vi "DriveControlLoop.vi"() -> ()   [LabVIEW 2018]
uses:
  <vilib>/Rock Robotics/WPI/ThirdParty/Phoenix-LabVIEW/Motor Controller/Controls/CTRE_Phoenix_MotorControl_ControlMode.ctl
  Infrastructure/RobotMap.vi
  Robot Global Data.vi
  <vilib>/Rock Robotics/WPI/ThirdParty/Phoenix-LabVIEW/Motor Controller/Get/CTRE_Phoenix_MotorController_GetQuadratureData.vi
panel:
  out "Motor Outupt":dbl[](graph)
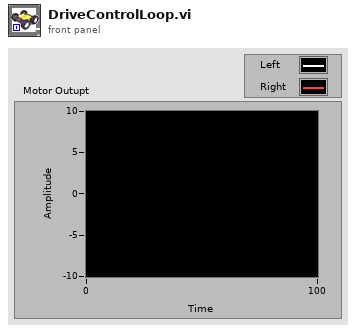
[diagram p1: front panel]
types:
  T1 = typedef "CTRE_Phoenix_MotorControl_ControlMode.ctl" = u16
  T2 = typedef "WPI_MotorControlDeviceRef.ctl" = cluster{"DeviceStatus":errorcluster, "Type":T3, "PWM":cluster{"PWM Channel":T4, "DeadBand":T5}, "CAN":cluster{"Device Number":u8, "SetOutput VI Ref":variant, "GetOutput VI Ref":variant, "Enable VI Ref":variant, "Disable VI Ref":variant, "Data":variant}, "Invert":bool, "DIO PWM":cluster{"PWM \"Enable\" Channel":T4, "DIOChannel":T6, "PWM Rate":dbl}}
  T3 = typedef "WPI_MotorControlType.ctl" = enum16{"PWM", "CAN", "DIO PWM"}
  T4 = typedef "FPGA_DIOPWMChannel.ctl" = enum8{"PWM 0", "PWM 1", "PWM 2", "PWM 3", "PWM 4", "PWM 5", "PWM 6", "PWM 7", "PWM 8", "PWM 9", "PWM MXP 0", "PWM MXP 1", "PWM MXP 2", "PWM MXP 3", "PWM MXP 4", "PWM MXP 5", "PWM MXP 6", "PWM MXP 7", "PWM MXP 8", "PWM MXP 9", "Invalid"}
  T5 = typedef "WPI_PWMDeadband.ctl" = cluster{"Name":string, "maxPositivePwm":i32, "minPositivePwm":i32, "centerPwm":i32, "maxNegativePwm":i32, "minNegativePwm":i32, "angularRange":u16}
  T6 = typedef "FPGA_DIOChannel.ctl" = enum8{"DIO 0", "DIO 1", "DIO 2", "DIO 3", "DIO 4", "DIO 5", "DIO 6", "DIO 7", "DIO 8", "DIO 9", "DIO MXP 0", "DIO MXP 1", "DIO MXP 2", "DIO MXP 3", "DIO MXP 4", "DIO MXP 5", "DIO MXP 6", "DIO MXP 7", "DIO MXP 8", "DIO MXP 9", "DIO MXP 10", "DIO MXP 11", "DIO MXP 12", "DIO MXP 13", "DIO MXP 14", "DIO MXP 15", "SPI Port CS1", "SPI Port CS2", "SPI Port CS3", "SPI Port MISO", "SPI Port MOSI", "Invalid"}
  T7 = typedef "WPI_DriverStationRobotMode2.ctl" = enum16{"Autonomous Disabled", "Autonomous Enabled", "Teleop Disabled", "Teleop Enabled", "Disconnected", "Finish", "Test Disabled", "Test Enabled", "Emergency Stopped"}
  T8 = typedef "Drive Motion Magic Setpoints.ctl" = cluster{"Increase in Left":dbl, "Increase in Right":dbl}[]
  T9 = cluster{"Increase in Left":dbl, "Increase in Right":dbl}
  T10 = typedef "Joystick Controls.ctl" = cluster{"Driver Left Joystick X":dbl, "Driver Left Joystick Y":dbl, "Driver A Button":bool, "Driver B Button":bool, "Driver X Button":bool, "Driver Y Button":bool, "Driver Left Bumper":bool, "Driver Right Bumper":bool, "Driver View Button":bool, "Driver Menu Button":bool, "Driver Left Joystick Press":bool, "Driver Right Joystick Press":bool, "Driver Left Trigger":dbl, "Driver Right Joystick X":dbl, "Driver Right Joystick Y":dbl, "Driver Right Trigger":dbl, "Operator Left Joystick X":dbl, "Operator Left Joystick Y":dbl, "Operator A Button":bool, "Operator B Button":bool, "Operator X Button":bool, "Operator Y Button":bool, "Operator Left Bumper":bool, "Operator Right Bumper":bool, "Operator View Button":bool, "Operator Menu Button":bool, "Operator Left Joystick Press":bool, "Operator Right Joystick Press":bool, "Operator Left Trigger":dbl, "Operator Right Joystick X":dbl, "Operator Right Joystick Y":dbl, "Operator Right Trigger":dbl, "Driver D-Pad":i16, "Operator D-Pad":i16}
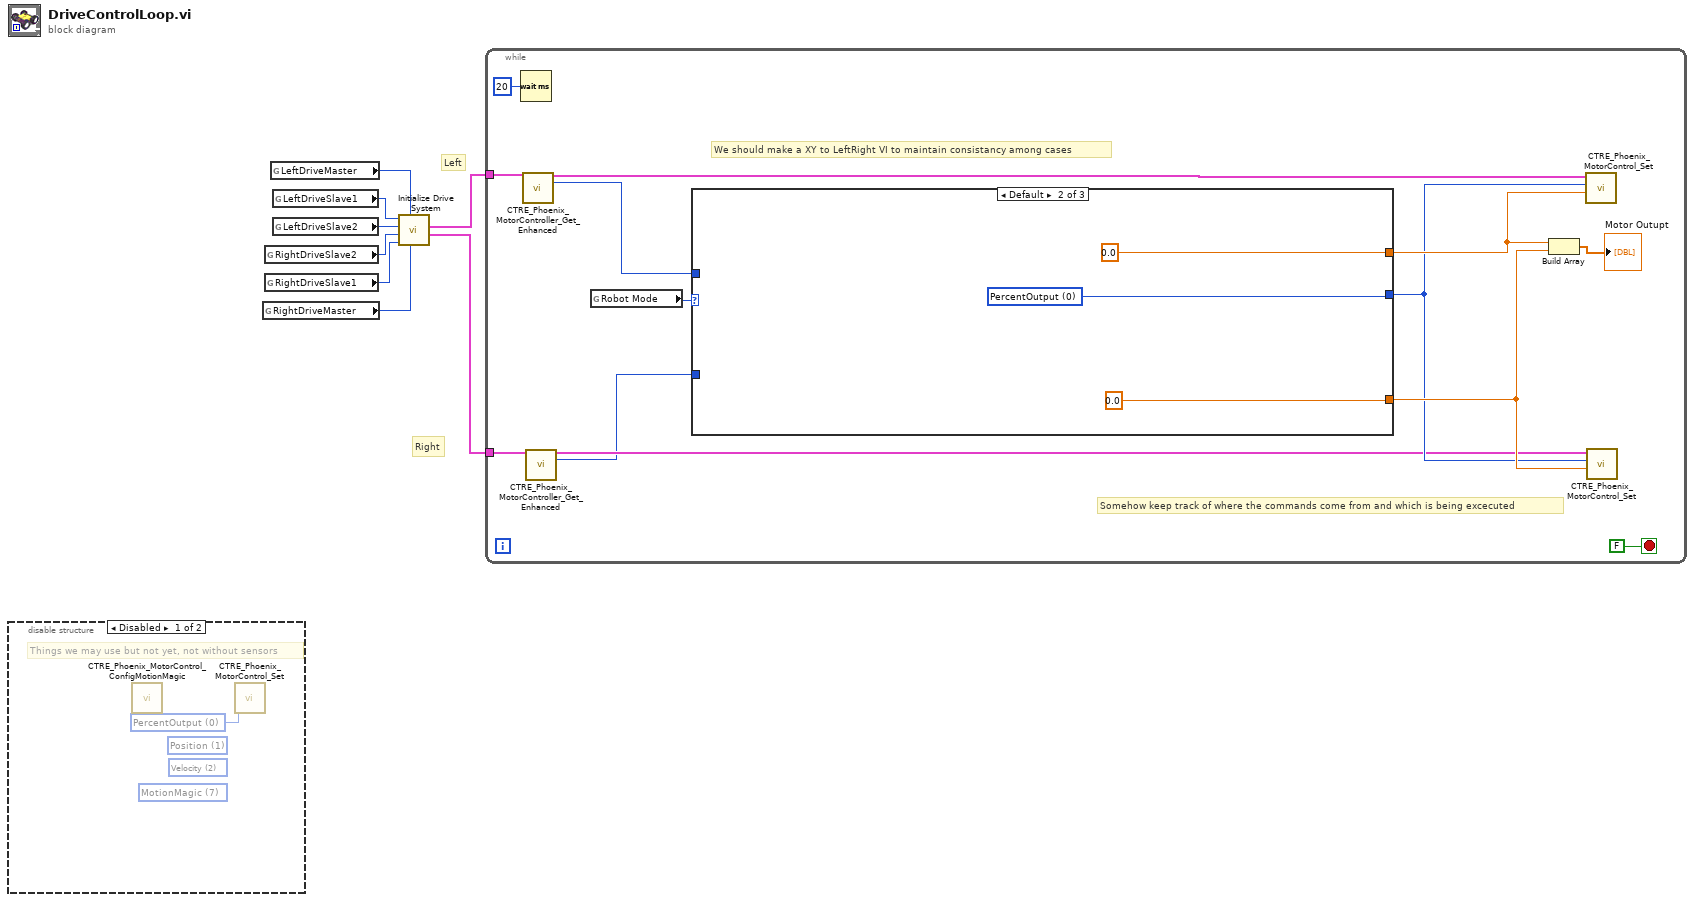
[diagram p0: block diagram]
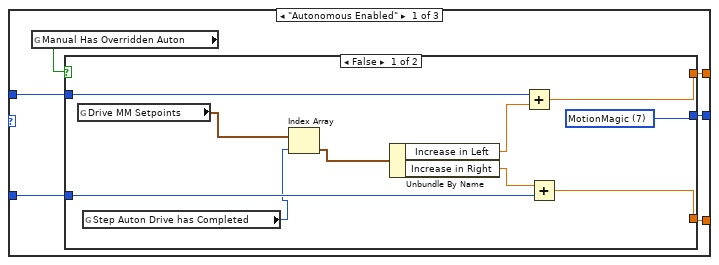
[diagram p3: hidden frame]
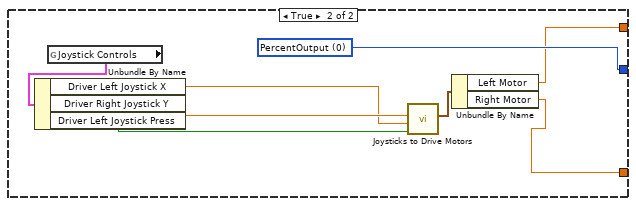
[diagram p4: hidden frame]
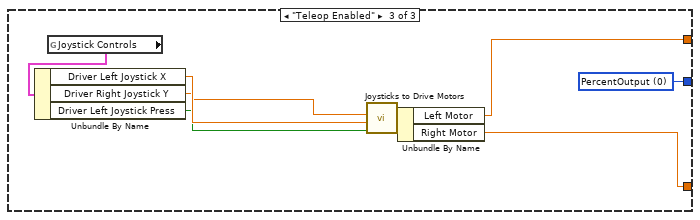
[diagram p5: hidden frame]
diagram:
  # "Right"
  # "Left"
  n1 = disable-structure shown="Disabled" {
    frame Disabled {
      (unwired) T1 7 items=["PercentOutput"=0, "Position"=1, "Velocity"=2, "Current"=3, "Follower"=5, "MotionProfile"=6, "MotionMagic"=7, "MotionProfileArc"=10, "Disabled"=15] ("Control Mode")
      (unwired) T1 2 items=["PercentOutput"=0, "Position"=1, "Velocity"=2, "Current"=3, "Follower"=5, "MotionProfile"=6, "MotionMagic"=7, "MotionProfileArc"=10, "Disabled"=15] ("Control Mode")
      (unwired) T1 1 items=["PercentOutput"=0, "Position"=1, "Velocity"=2, "Current"=3, "Follower"=5, "MotionProfile"=6, "MotionMagic"=7, "MotionProfileArc"=10, "Disabled"=15] ("Control Mode")
      w9 = T1 0 items=["PercentOutput"=0, "Position"=1, "Velocity"=2, "Current"=3, "Follower"=5, "MotionProfile"=6, "MotionMagic"=7, "MotionProfileArc"=10, "Disabled"=15] ("Control Mode")
      # "Things we may use but not yet, not without sensors"
      n2 = call <vilib>:"CTRE_Phoenix_MotorControl_ConfigMotionMagic.vi"() -> ()  [unwired: 10 in, 2 out]
      n3 = call <vilib>:"CTRE_Phoenix_MotorControl_Set.vi"("Control Mode"=w9) -> ()  [unwired: 9 in, 2 out]
    }
    frame Enabled {
    }
  }
  n4 = global read "RobotMap.vi" "RightDriveMaster"() -> (w6:u8)
  n5 = global read "RobotMap.vi" "RightDriveSlave2"() -> (w8:u8)
  n6 = global read "RobotMap.vi" "RightDriveSlave1"() -> (w7:u8)
  n7 = global read "RobotMap.vi" "LeftDriveMaster"() -> (w3:u8)
  n8 = global read "RobotMap.vi" "LeftDriveSlave1"() -> (w4:u8)
  n9 = global read "RobotMap.vi" "LeftDriveSlave2"() -> (w5:u8)
  n10 = call "Initialize Drive System.vi"("RightDriveMaster"=w6, "LeftDriveMaster"=w3, "RightDriveSlave1"=w7, "RightDriveSlave2"=w8, "LeftDriveSlave 2"=w5, "LeftDriveSlave1"=w4) -> ("RightDriveMaster"=w1:T2, "LeftDriveMaster"=w2:T2)  [unwired: 4 in]
  n11 = while {
    tunnel: w2 -> [w15]
    tunnel: w1 -> [w13]
    stop <- FALSE stop-if-true
    # "We should make a XY to LeftRight VI to maintain consistancy among cases"
    # "Somehow keep track of where the commands come from and which is being excecuted"
    n12 = Wait (ms)(milliseconds to wait=u32 20) -> ()  [unwired: 1 out]
    n13 = call-poly <vilib>:"CTRE_Phoenix_MotorController_Get_Enhanced.vi"("PhoenixMotorControlDevRef"=w15) -> ("PhoenixMotorControlDevRef"=w14:T2, "Quadrature Position"=w11:i32)  [unwired: 11 in, 2 out]
    n14 = call-poly <vilib>:"CTRE_Phoenix_MotorController_Get_Enhanced.vi"("PhoenixMotorControlDevRef"=w13) -> ("PhoenixMotorControlDevRef"=w12:T2, "Quadrature Position"=w10:i32)  [unwired: 11 in, 2 out]
    n15 = global read "Robot Global Data.vi" "Robot Mode"() -> (w19:T7)
    n16 = case shown="Default" w19 {
      tunnel: [w27 0.0 ("Left Motor Value") w51] -> w17
      tunnel: [w25 0.0 ("Left Motor Value") w50] -> w18
      tunnel: [w26 w49 w56] -> w16
      tunnel: w11 -> [w24 _ _]
      tunnel: w10 -> [w23 _ _]
      frame "Autonomous Enabled" {
        n17 = global read "Robot Global Data.vi" "Manual Has Overridden Auton"() -> (w28:bool)
        n18 = case shown="False" w28 {
          tunnel: [w37 w39] -> w27
          tunnel: [w36 w40] -> w25
          tunnel: [w38 w45] -> w26
          tunnel: w24 -> [w35 _]
          tunnel: w23 -> [w34 _]
          frame False {
            w38 = T1 7 items=["PercentOutput"=0, "Position"=1, "Velocity"=2, "Current"=3, "Follower"=5, "MotionProfile"=6, "MotionMagic"=7, "MotionProfileArc"=10, "Disabled"=15] ("Control Mode")
            n19 = global read "Robot Global Data.vi" "Drive MM Setpoints"() -> (w32:T8)
            n20 = global read "Robot Global Data.vi" "Step Auton Drive has Completed"() -> (w33:i32)
            n21 = Index Array(array=w32, index=w33) -> (element=w31:T9)
            n22 = Unbundle By Name(w31) -> ("Increase in Left"=w30:dbl, "Increase in Right"=w29:dbl)
            n23 = Add(x=w35, y=w30) -> (x+y=w37:dbl)
            n24 = Add(x=w29, y=w34) -> (x+y=w36:dbl)
          }
          frame True {
            w45 = T1 0 items=["PercentOutput"=0, "Position"=1, "Velocity"=2, "Current"=3, "Follower"=5, "MotionProfile"=6, "MotionMagic"=7, "MotionProfileArc"=10, "Disabled"=15] ("Control Mode")
            n25 = global read "Robot Global Data.vi" "Joystick Controls"() -> (w46:T10)
            n26 = Unbundle By Name(w46) -> ("Driver Left Joystick X"=w43:dbl, "Driver Right Joystick Y"=w44:dbl, "Driver Left Joystick Press"=w42:bool)
            n27 = call "Joysticks to Drive Motors.vi"("Boost?"=w42, "Turn"=w43, "Throttle"=w44) -> ("Drive Motor Values"=w41:cluster{"Left Motor":dbl, "Right Motor":dbl})  [unwired: 8 in]
            n28 = Unbundle By Name(w41) -> ("Left Motor"=w39:dbl, "Right Motor"=w40:dbl)
          }
        }
      }
      frame Default {
        w49 = T1 0 items=["PercentOutput"=0, "Position"=1, "Velocity"=2, "Current"=3, "Follower"=5, "MotionProfile"=6, "MotionMagic"=7, "MotionProfileArc"=10, "Disabled"=15] ("Control Mode")
      }
      frame "Teleop Enabled" {
        w56 = T1 0 items=["PercentOutput"=0, "Position"=1, "Velocity"=2, "Current"=3, "Follower"=5, "MotionProfile"=6, "MotionMagic"=7, "MotionProfileArc"=10, "Disabled"=15] ("Control Mode")
        n29 = global read "Robot Global Data.vi" "Joystick Controls"() -> (w57:T10)
        n30 = Unbundle By Name(w57) -> ("Driver Left Joystick X"=w55:dbl, "Driver Right Joystick Y"=w54:dbl, "Driver Left Joystick Press"=w53:bool)
        n31 = call "Joysticks to Drive Motors.vi"("Boost?"=w53, "Turn"=w55, "Throttle"=w54) -> ("Drive Motor Values"=w52:cluster{"Left Motor":dbl, "Right Motor":dbl})  [unwired: 8 in]
        n32 = Unbundle By Name(w52) -> ("Left Motor"=w51:dbl, "Right Motor"=w50:dbl)
      }
    }
    n33 = Build Array(w17, w18) -> (→"Motor Outupt":dbl[])
    n34 = call <vilib>:"CTRE_Phoenix_MotorControl_Set.vi"("Output"=w17, "Control Mode"=w16, "PhoenixMotorControlDevRef"=w14) -> ()  [unwired: 7 in, 2 out]
    n35 = call <vilib>:"CTRE_Phoenix_MotorControl_Set.vi"("Output"=w18, "Control Mode"=w16, "PhoenixMotorControlDevRef"=w12) -> ()  [unwired: 7 in, 2 out]
  }
